vi "Configure the Test OK Message.vi"(5 "Query the Message":bool, 7 "Setup the Message":bool, 8 "error in":errorcluster, 10 "Send Message when test stop":u8(ring) items=["OFF", "ON"], 11 "VISA resource name":refnum<visa-resource-name>) -> (0 "error out":errorcluster, 2 "Return the Send Message Status":string, 3 "VISA resource name out":refnum<visa-resource-name>)   [LabVIEW 2021, in "GPT-9000.lvlib"]
uses:
  GPT-9000.lvlib
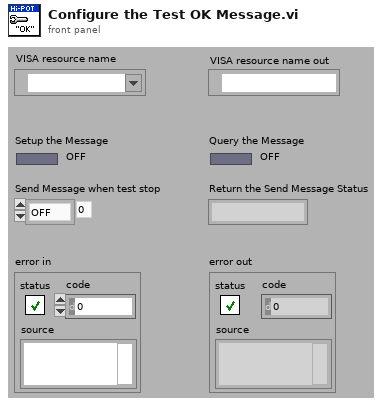
[diagram p1: front panel]
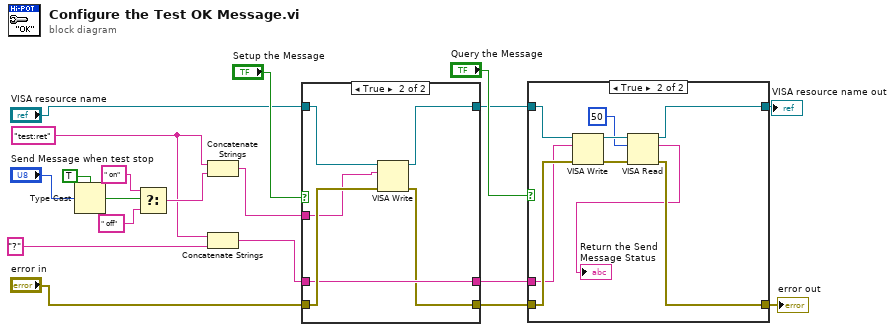
[diagram p0: block diagram]
diagram:
  w12 = "test:ret"
  n1 = Type Cast(type=TRUE, x="Send Message when test stop") -> (*(type *) &x=w17:bool)
  n2 = Select(t=" on", s=w17, f=" off") -> (s? t:f=w14:string)
  n3 = Concatenate Strings(w12, w14) -> (w10:string)
  n4 = Concatenate Strings(w12, "?") -> (w9:string)
  n5 = case shown="True" "Setup the Message" {
    tunnel: w10 -> [_ w26]
    tunnel: w9 -> [w22 w25]
    tunnel: [w22 w25] -> w3
    tunnel: "VISA resource name" -> [w21 w28]
    tunnel: [w21 w24] -> w5
    tunnel: "error in" -> [w20 w27]
    tunnel: [w20 w23] -> w4
    frame False {
    }
    frame True {
      n6 = VISA Write(VISA resource name=w28, write buffer=w26, error in (no error)=w27) -> (VISA resource name out=w24:refnum<visa-resource-name>, error out=w23:errorcluster)  [unwired: 1 out]
    }
  }
  n7 = case shown="True" "Query the Message" {
    tunnel: w5 -> [w30 w36]
    tunnel: w4 -> [w29 w35]
    tunnel: w3 -> [_ w34]
    tunnel: [w30 w33] -> w2
    tunnel: [w29 w32] -> w1
    frame False {
    }
    frame True {
      n8 = VISA Write(VISA resource name=w36, write buffer=w34, error in (no error)=w35) -> (VISA resource name out=w38:refnum<visa-resource-name>, error out=w39:errorcluster)  [unwired: 1 out]
      n9 = VISA Read(VISA resource name=w38, byte count=u32 50, error in (no error)=w39) -> (VISA resource name out=w33:refnum<visa-resource-name>, read buffer=→"Return the Send Message Status":string, error out=w32:errorcluster)  [unwired: 1 out]
    }
  }
  "VISA resource name out" <- w2
  "error out" <- w1
